vi "autoGearGrabber.vi"(8 "error in (no error)":errorcluster, 10 "gear":string="gear", 11 "drive":string="RobotDrive") -> (0 "error out":errorcluster)   [LabVIEW 2016]
uses:
  <vilib>/Rock Robotics/WPI/Utilities/WPI_GetSetVariantRefNum.vi
  Auto.vi
  Accordian/placed.vi
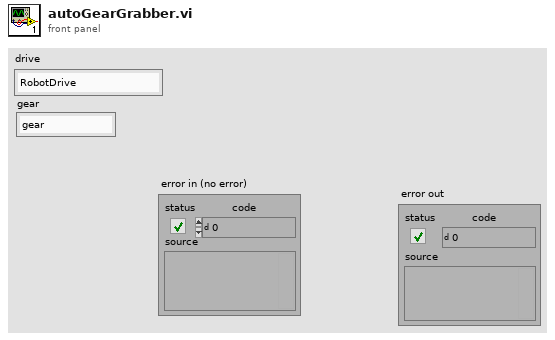
[diagram p1: front panel]
types:
  T1 = typedef "WPI_ServoDeviceRef.ctl" = cluster{"DeviceStatus":errorcluster, "PWM Channel":T2, "DeadBand":T3}
  T2 = typedef "FPGA_DIOPWMChannel.ctl" = enum8{"PWM 0", "PWM 1", "PWM 2", "PWM 3", "PWM 4", "PWM 5", "PWM 6", "PWM 7", "PWM 8", "PWM 9", "PWM MXP 0", "PWM MXP 1", "PWM MXP 2", "PWM MXP 3", "PWM MXP 4", "PWM MXP 5", "PWM MXP 6", "PWM MXP 7", "PWM MXP 8", "PWM MXP 9", "Invalid"}
  T3 = typedef "WPI_PWMDeadband.ctl" = cluster{"Name":string, "maxPositivePwm":i32, "minPositivePwm":i32, "centerPwm":i32, "maxNegativePwm":i32, "minNegativePwm":i32, "angularRange":u16}
  T4 = typedef "WPI_RobotDriveDevRef.ctl" = cluster{"DevStatus":errorcluster, "Motors[]":T5[], "Square Inputs":bool, "Max Output":dbl}
  T5 = typedef "WPI_MotorControlDeviceRef.ctl" = cluster{"DeviceStatus":errorcluster, "Type":T6, "PWM":cluster{"PWM Channel":T2, "DeadBand":T3}, "CAN":cluster{"Device Number":u8, "SetOutput VI Ref":variant, "GetOutput VI Ref":variant, "Enable VI Ref":variant, "Disable VI Ref":variant, "Data":variant}, "Invert":bool}
  T6 = typedef "WPI_MotorControlType.ctl" = enum16{"PWM", "CAN"}
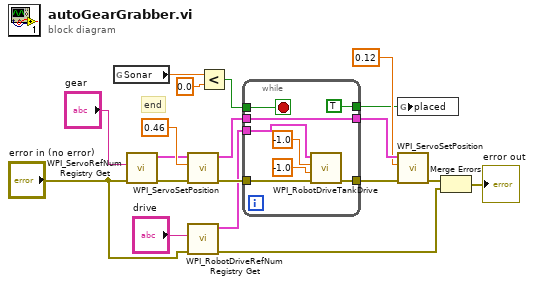
[diagram p0: block diagram]
diagram:
  # "end"
  n1 = global read "Auto.vi" "Sonar"() -> (w10:dbl)
  n2 = call <vilib>:"WPI_ServoRefNum Registry Get.vi"("error in (no error)"="error in (no error)", "refnum name"="gear") -> ("error out"=w16:errorcluster, "ServoDeviceRef"=w17:T1)  [unwired: 8 in]
  n3 = call <vilib>:"WPI_ServoSetPosition.vi"("error in (no error)"=w16, "Position"=0.46, "ServoDeviceRef"=w17) -> ("error out"=w14:errorcluster, "ServoDeviceRef"=w6:T1)  [unwired: 7 in]
  n4 = call <vilib>:"WPI_RobotDriveRefNum Registry Get.vi"("error in (no error)"="error in (no error)", "refnum name"="drive") -> ("error out"=w3:errorcluster, "RobotDriveDevRef"=w13:T4)  [unwired: 8 in]
  n5 = Less?(x=w10, y=0.0) -> (x < y?=w8:bool)
  n6 = while {
    tunnel: w14 -> [w25]
    tunnel: w13 -> [w24]
    tunnel: w8 -> [w23]
    tunnel: [w22] -> w7
    tunnel: w6 -> [w22]
    tunnel: [w21] -> w5
    tunnel: [TRUE ("placed")] -> w2
    stop <- w23 stop-if-true
    n7 = call <vilib>:"WPI_RobotDriveTankDrive.vi"("error in (no error)"=w25, "Right axis value"=-1.0, "Left axis value"=-1.0, "RobotDriveDevRef"=w24) -> ("error out"=w21:errorcluster)  [unwired: 5 in, 2 out]
  }
  n8 = global write "placed.vi" "placed"(w2) -> ()
  n9 = call <vilib>:"WPI_ServoSetPosition.vi"("error in (no error)"=w5, "Position"=0.12, "ServoDeviceRef"=w7) -> ("error out"=w1:errorcluster)  [unwired: 7 in, 1 out]
  n10 = Merge Errors(w1, w3) -> (→"error out":errorcluster)
